vi "gfitsio-check-valid-refnum.vi"(4 "gftis refnum":T1) -> (1 "invalid refnum?":bool)   [LabVIEW 2019, in "gfitsio.lvlib"]
doc: "Returns TRUE if <B>gftis refnum</B> is invalid. Use this function to make sure a reference to a file still resides in system memory and was not closed."
uses:
  gfitsio.lvlib
  gfitsio-refnum.ctl
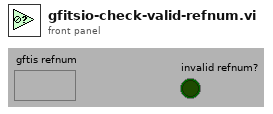
[diagram p1: front panel]
types:
  T1 = typedef "gfitsio.lvlib/gfitsio-refnum.ctl" = refnum<k1>
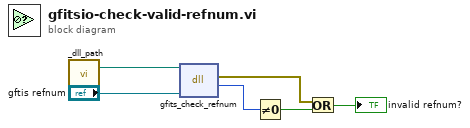
[diagram p0: block diagram]
diagram:
  n1 = call "_dll_path.vi"() -> ("Path"=w4:path)  [unwired: 1 in]
  n2 = dll-call lib="?" fn="gfits_check_refnum"(path in=w4, "refnum"="gftis refnum") -> (error out=w2:errorcluster, "return type"=w6:i32)  [unwired: 3 in, 1 out]
  n3 = Not Equal To 0?(x=w6) -> (x != 0?=w3:bool)
  n4 = Or(x=w2, y=w3) -> (x .or. y?=→"invalid refnum?":bool)
